vi "DriveTest.vi"() -> ()   [LabVIEW 2009]
uses:
  Drive.lvlib
  FPGA.lvlib
  Motor.lvlib
panel:
  in  "stop":bool
  in  "Y_Speed":dbl(slide) min=-1.0 max=1.0 scale=-1.0..1.0
  in  "X_Speed":dbl(slide) min=-1.0 max=1.0 scale=-1.0..1.0
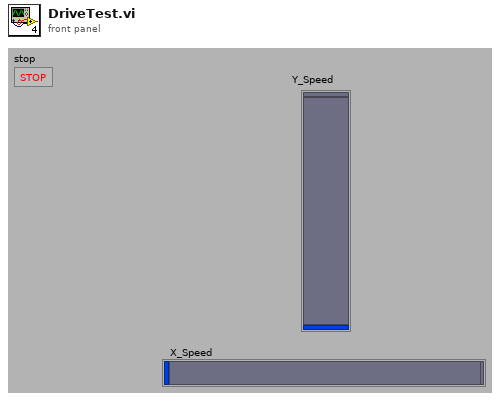
[diagram p1: front panel]
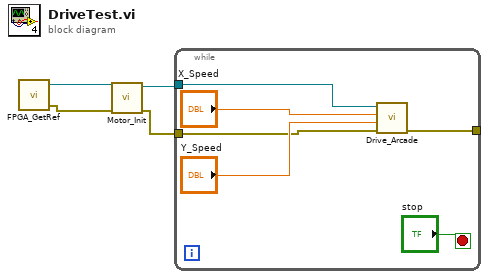
[diagram p0: block diagram]
diagram:
  n1 = call "FPGA_GetRef.vi"() -> ("error out"=w3:errorcluster, "FPGA_Ref"=w4:refnum<k20>)  [unwired: 1 in]
  n2 = call "Motor_Init.vi"("error in"=w3, "FPGA_Ref_in"=w4) -> ("error out"=w1:errorcluster, "FPGA_Ref_out"=w2:refnum<k20>)  [unwired: 8 in]
  n3 = while {
    tunnel: [w7] -> _
    tunnel: w2 -> [w6]
    tunnel: w1 -> [w5]
    stop <- "stop" stop-if-true
    n4 = call "Drive_Arcade.vi"("error in"=w5, "Y_Speed"="Y_Speed", "X_Speed"="X_Speed", "FPGA_Ref_in"=w6) -> ("error out"=w7:errorcluster)  [unwired: 7 in]
  }
